vi "piezoAutofocus.vi"(1 "piezoStep":dbl, 2 "volumeIn":u16[][][](array[numeric])) -> (0 "moved piezo":bool)   [LabVIEW 2017]
uses:
  globalDevices.vi
  <vilib>/Analysis/baseanly.llb/Std Deviation and Variance.vi
  globalUtilities.vi
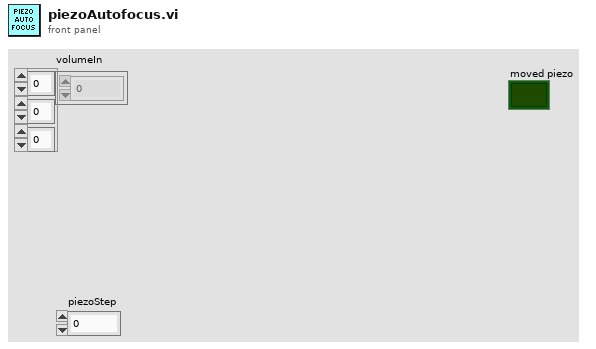
[diagram p1: front panel]
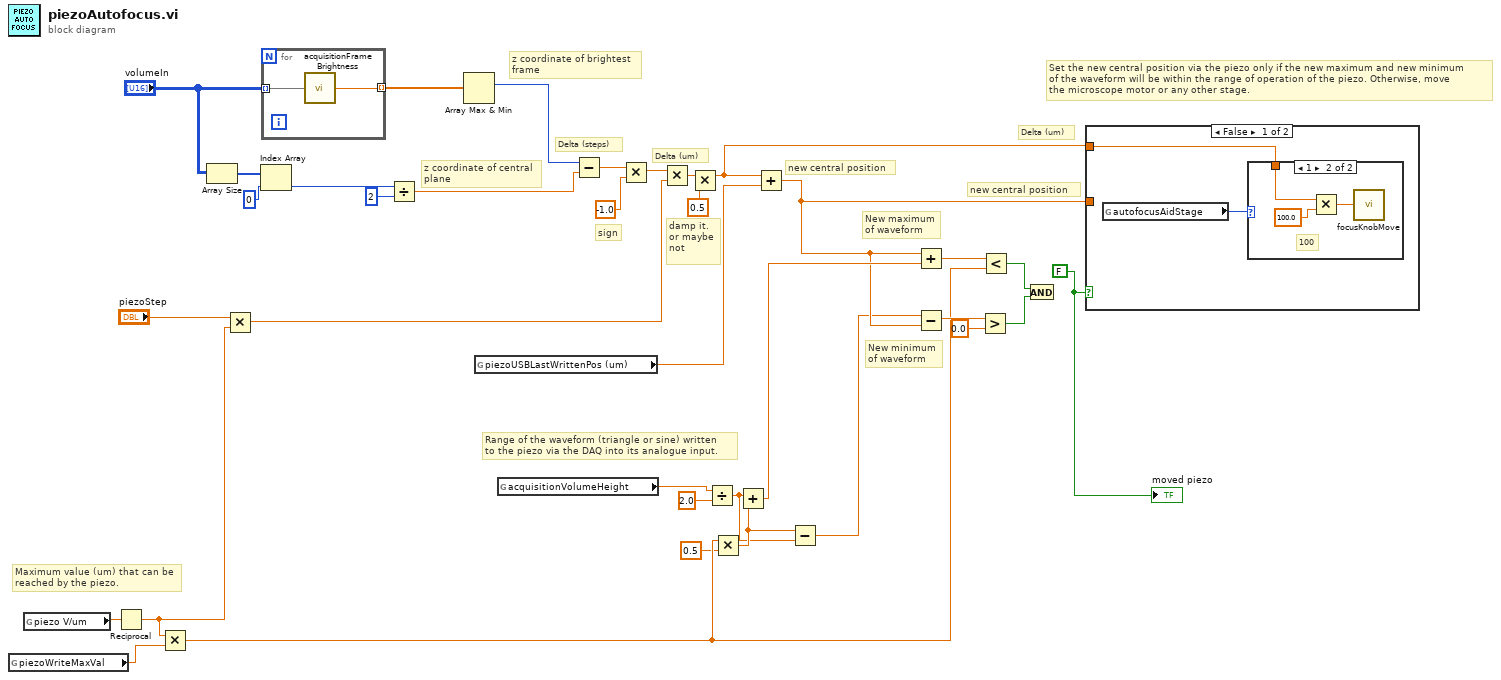
[diagram p0: block diagram]
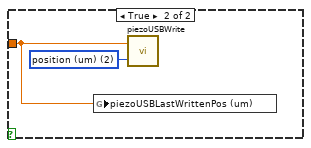
[diagram p3: hidden frame]
diagram:
  w1 = FALSE
  # "sign"
  # "damp it.\nor maybe\nnot"
  # "Delta (um)"
  # "new central position"
  # "Maximum value (um) that can be\nreached by the piezo."
  # "z coordinate of central\nplane"
  # "z coordinate of brightest\nframe"
  # "Set the new central position via the piezo only if the new maximum and new minimum\nof the waveform will be within the range of operation of the piezo. Otherwise, move\nthe microscope motor or any other stage."
  # "New minimum\nof waveform"
  # "New maximum\nof waveform"
  # "Range of the waveform (triangle or sine) written\nto the piezo via the DAQ into its analogue input."
  # "Delta (um)"
  # "Delta (steps)"
  # "new central position"
  n1 = global read "globalDevices.vi" "piezoWriteMaxVal"() -> (w22:dbl)
  n2 = global read "globalDevices.vi" "piezo V/um"() -> (w23:dbl)
  n3 = Reciprocal(x=w23) -> (1/x=w7:dbl)
  n4 = Multiply(x=w7, y=w22) -> (x*y=w16:dbl)
  n5 = Array Size(array="volumeIn") -> (size(s)=w34:i32[])
  n6 = Multiply(x="piezoStep", y=w7) -> (x*y=w9:dbl)
  n7 = Index Array(array=w34, index=0) -> (element=w19:i32)
  n8 = for {
    tunnel: "volumeIn" -> [w37] mode=indexing
    tunnel: [w36] -> w10 mode=indexing
    n9 = call "acquisitionFrameBrightness.vi"("frame"=w37) -> ("brighness"=w36:dbl)
  }
  n10 = Divide(x=w19, y=2) -> (x/y=w17:dbl)
  n11 = Array Max & Min(array=w10) -> (max index (indices)=w32:i32)  [unwired: 3 out]
  n12 = global read "globalDevices.vi" "piezoUSBLastWrittenPos (um)"() -> (w29:dbl)
  n13 = global read "globalUtilities.vi" "acquisitionVolumeHeight"() -> (w28:dbl)
  n14 = Subtract(x=w32, y=w17) -> (x-y=w31:dbl)
  n15 = Multiply(x=w31, y=-1.0) -> (x*y=w30:dbl)
  n16 = Multiply(x=w30, y=w9) -> (x*y=w14:dbl)
  n17 = Multiply(x=w14, y=0.5) -> (x*y=w13:dbl)
  n18 = Divide(x=w28, y=2.0) -> (x/y=w2:dbl)
  n19 = Multiply(x=w16, y=0.5) -> (x*y=w3:dbl)
  n20 = Add(x=w2, y=w3) -> (x+y=w6:dbl)
  n21 = Add(x=w13, y=w29) -> (x+y=w5:dbl)
  n22 = Subtract(x=w3, y=w2) -> (x-y=w4:dbl)
  n23 = Add(x=w5, y=w6) -> (x+y=w24:dbl)
  n24 = Subtract(x=w4, y=w5) -> (x-y=w26:dbl)
  n25 = Greater?(x=w26, y=0.0) -> (0:w20:bool)
  n26 = Less?(x=w24, y=w16) -> (x < y?=w21:bool)
  n27 = And(x=w21, y=w20) -> ()  [unwired: 1 out]
  n28 = case shown="False" w1 {
    tunnel: w5 -> [_ w43]
    tunnel: w13 -> [w39 _]
    frame False {
      n29 = global read "globalDevices.vi" "autofocusAidStage"() -> (w38:u16)
      n30 = case shown="1" w38 {
        tunnel: w39 -> [_ w42]
        frame 0, Default {
          # "None."
        }
        frame 1 {
          # "100"
          n31 = Multiply(x=w42, y=100.0) -> (x*y=w40:dbl)
          n32 = call "focusKnobMove.vi"("position (10^-4 m)"=w40) -> ()  [unwired: 1 in]
        }
      }
    }
    frame True {
      w44 = u16 2 items=["fractional", "voltage (V)", "position (um)"] ("mode")
      n33 = global write "globalDevices.vi" "piezoUSBLastWrittenPos (um)"(w43) -> ()
      n34 = call "piezoUSBWrite.vi"("mode"=w44, "position"=w43) -> ()  [unwired: 1 in]
    }
  }
  "moved piezo" <- w1
